vi "To File (Ref).vi"(6 "Pretty Print?":bool=TRUE, 7 "enable LabVIEW extensions? (T)":bool=TRUE, 8 "error in (no error)":errorcluster, 10 "JSON Value in":variant, 11 "refnum in":refnum<file>) -> (0 "error out":errorcluster, 3 "refnum out":refnum<file>)   [LabVIEW 2017, in "Advanced Variant Tools.lvlib" / "JSON.lvlib"]
doc: "Saves a JSON instance's data to the given file."
uses:
  JSON/JSON.lvlib
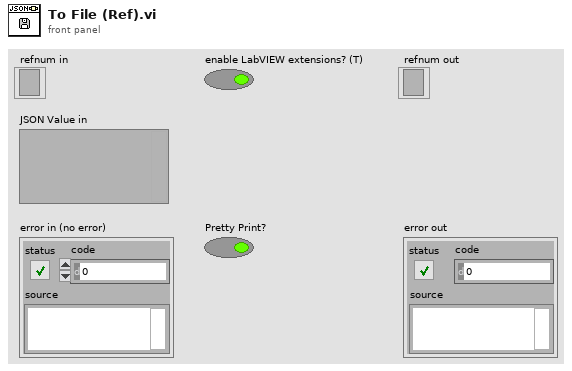
[diagram p1: front panel]
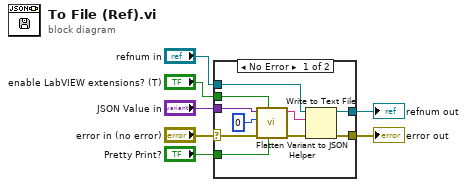
[diagram p0: block diagram]
diagram:
  n1 = case shown="No Error" "error in (no error)" {
    selector: "error in (no error)" -> [w15 w19]
    tunnel: "JSON Value in" -> [w17 _]
    tunnel: [w12 w19] -> w5
    tunnel: "Pretty Print?" -> [w10 _]
    tunnel: "refnum in" -> [w13 w18]
    tunnel: [w11 w18] -> w2
    tunnel: "enable LabVIEW extensions? (T)" -> [w9 _]
    frame No Error {
      n2 = call "Flatten Variant to JSON Helper.vi"("pretty print? (T)"=w10, "enable LabVIEW extensions? (T)"=w9, "error in (no error)"=w15, "indent"=0, "JSON Value in"=w17) -> ("error out"=w14:errorcluster, "String"=w16:string)  [unwired: 5 in]
      n3 = Write to Text File(file (use dialog)=w13, text=w16, error in=w14) -> (refnum out=w11:refnum<file>, error out=w12:errorcluster)  [unwired: 1 in, 1 out]
    }
    frame Error {
    }
  }
  "error out" <- w5
  "refnum out" <- w2
